vi "Facade.vi"(0 "Data In":T8, 2 "Display State In":T2, 3 "Container State":T7) -> (6 "Data Out":T8, 7 "Display State Out":T2, 8 "Action":T1)   [LabVIEW 2020, in "Interactive Graph.xctl"]
uses:
  Interactive Graph.xctl
  Data.vi
  EPhys/LV Source/Work Panel VIs/Typedefs/EPhysWork-Label Position.ctl
  <vilib>/_xctls/Container State.ctl
  State.vi
  Persistent.ctl
  Plot.ctl
  Events.ctl
  Selection.ctl
  XRange.ctl
  YScale.ctl
  Cursor.ctl
  <vilib>/_xctls/Action.ctl
  Scale Selector/Scale Selector.xctl
  <vilib>/Utility/miscctls.llb/LVAnnotationListTypeDef.ctl
  <vilib>/_xctls/XControlSupport.lvlib
panel:
  in  "Scale":dbl(xcontrol)
  out "Graph":cluster{dbl[], dbl[]}[](graph)
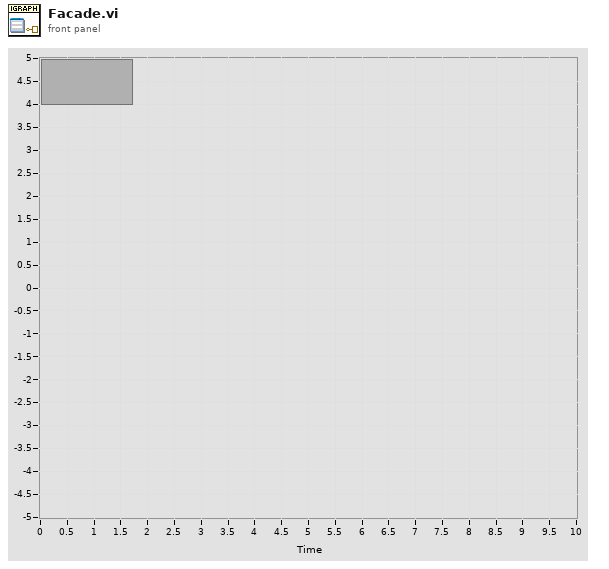
[diagram p1: front panel]
types:
  T1 = typedef "XControlSupport.lvlib/Action.ctl" = cluster{"Data Changed?":bool, "State Changed?":bool, "Action Name":string}
  T2 = typedef "Interactive Graph.xctl/State.vi" = cluster{"ref":refnum<vi>, "actions":string[], "Persist":T3, "cursor":bool, "prescale":dbl, "palette":u32[], "colIndex":i32, "to add":T4, "Events":T6, "selected":i32, "to show":cluster{"Visible":bool, "Start":i32, "Length":i32}, "maxplot":i32, "Y0":dbl[], "plotnum":i32, "length":i32}
  T3 = typedef "Interactive Graph.xctl/Persistent.ctl" = cluster{"Scale":dbl, "Xrange":cluster{"min":dbl, "max":dbl}}
  T4 = typedef "Interactive Graph.xctl/Plot.ctl" = cluster{"plot":cluster{"X":dbl[], "Y":dbl[]}, "name":string, "Y0":dbl, "color":u32, "Style":enum16{"Normal", "Highlight", "Shadow"}, "labpos":T5, "visible":bool, "cursor":bool}
  T5 = typedef "EPhysWork-Label Position.ctl" = cluster{"Index":i32, "Xoff":dbl, "Yoff":dbl}
  T6 = typedef "Interactive Graph.xctl/Events.ctl" = cluster{"Selection":refnum<user-event>, "XRange":refnum<user-event>, "YScale":refnum<user-event>, "CursorPos":refnum<user-event>}
  T7 = typedef "XControlSupport.lvlib/Container State.ctl" = cluster{"Indicator?":bool, "Run Mode?":bool, " Refnum":refnum<vi>}
  T8 = typedef "Interactive Graph.xctl/Data.vi" = cluster{"plot":cluster{"X":dbl[], "Y":dbl[]}, "name":string, "Y0":dbl, "color":u32, "Style":enum16{"Normal", "Highlight", "Shadow"}, "labpos":T5, "visible":bool, "cursor":bool}[]
  T9 = typedef "LVAnnotationListTypeDef.ctl" = cluster{"Name":string, "Color":u32, "Style":u8, "Point Style":u8, "Name Visible":bool, "Allow Drag":bool, "Annotation Mode":u32, "Plot":i32, "Index":i32, "Position":cluster{"X":dbl, "Y":dbl}, "X Scale":u32, "Y Scale":u32, "Show Arrow":bool, "Lock Name":bool, "Plot Area":i32, "Label Offset":cluster{"X":dbl, "Y":dbl}}[]
  T10 = typedef "LVRectTypeDef.ctl" = cluster{"Left":i16, "Top":i16, "Right":i16, "Bottom":i16}
  T11 = typedef "LVPoint32TypeDef.ctl" = cluster{"Horizontal":i32, "Vertical":i32}
  T12 = typedef "PlotDrag-State.ctl" = cluster{"PlotNum":i32, "Y0":dbl, "Plot":cluster{dbl[], dbl[]}, "Drag":bool, "Moved":bool, "dY":dbl, "keyIndex":i32}
  T13 = cluster{"plot":cluster{"X":dbl[], "Y":dbl[]}, "name":string, "Y0":dbl, "color":u32, "Style":enum16{"Normal", "Highlight", "Shadow"}, "labpos":T5, "visible":bool, "cursor":bool}[]
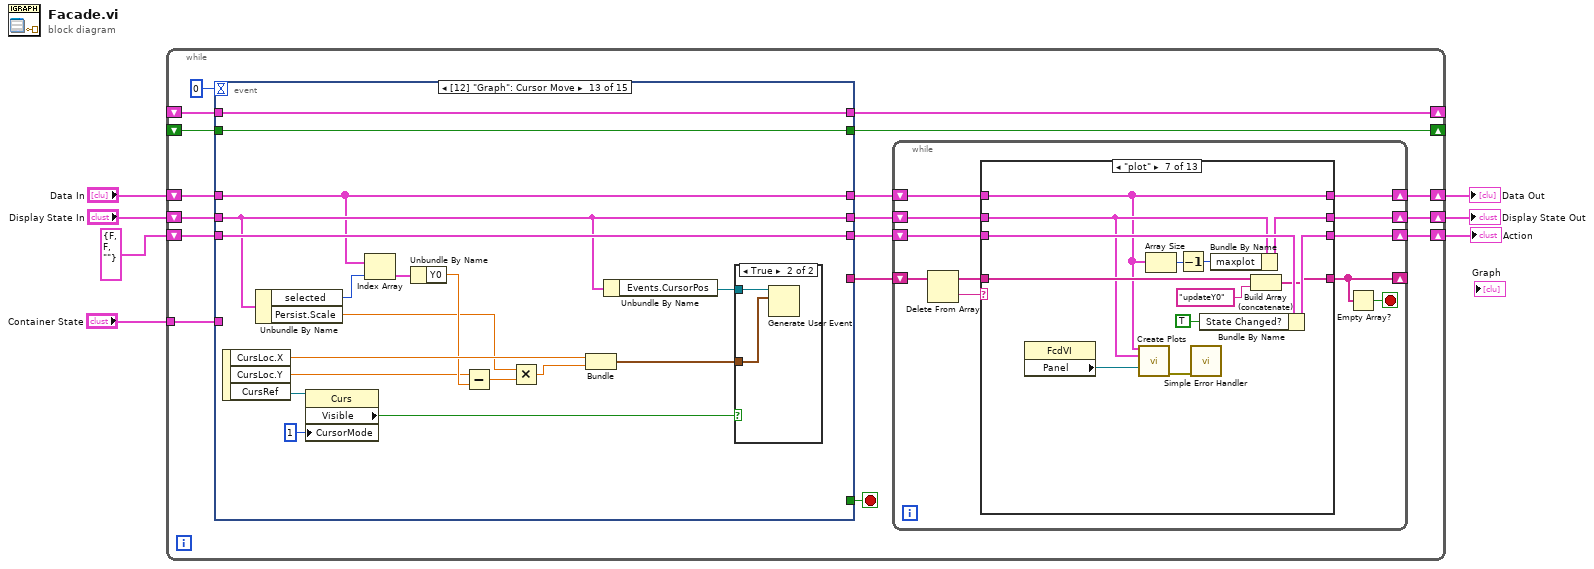
[diagram p0: block diagram]
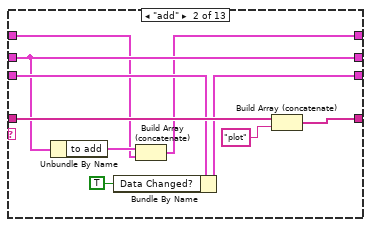
[diagram p3: hidden frame]
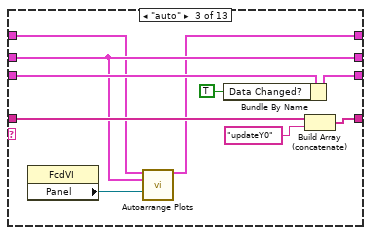
[diagram p4: hidden frame]
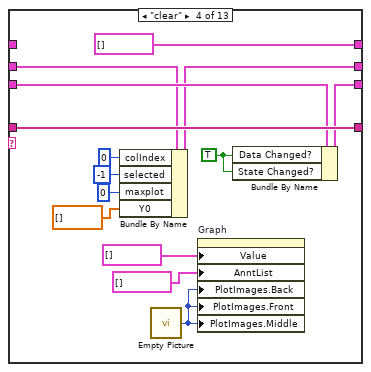
[diagram p5: hidden frame]
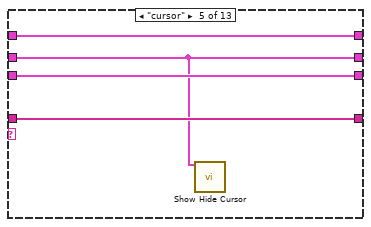
[diagram p6: hidden frame]
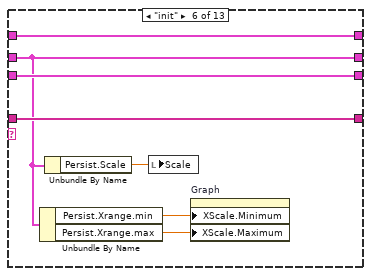
[diagram p7: hidden frame]
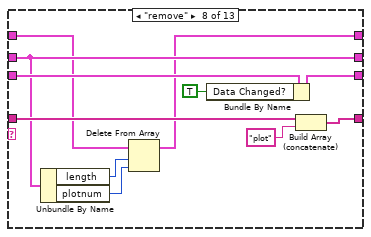
[diagram p8: hidden frame]
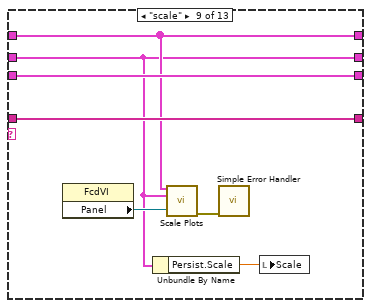
[diagram p9: hidden frame]
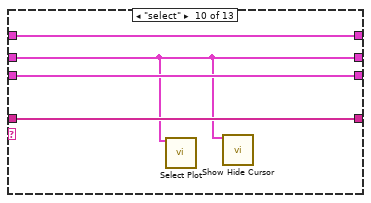
[diagram p10: hidden frame]
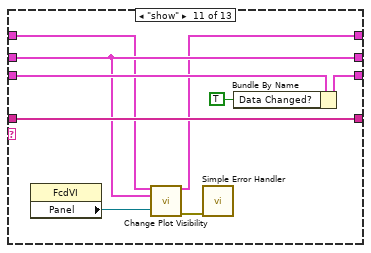
[diagram p11: hidden frame]
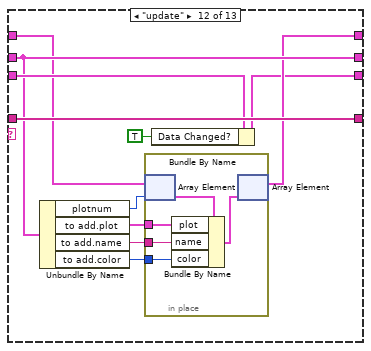
[diagram p12: hidden frame]
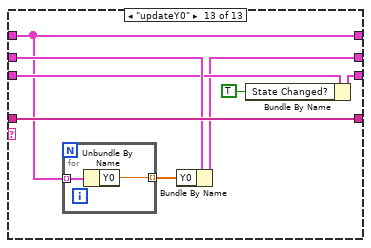
[diagram p13: hidden frame]
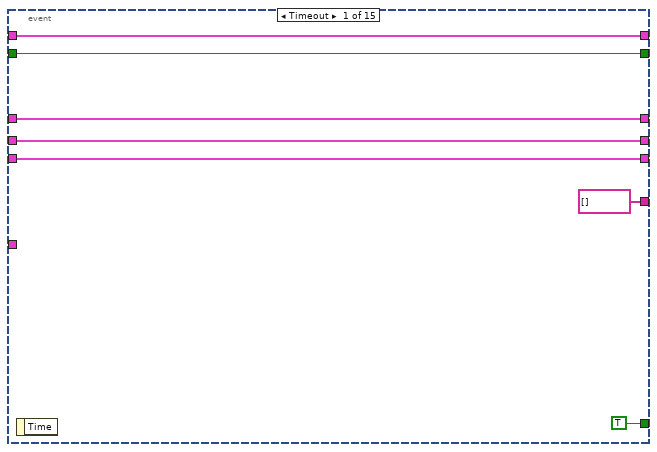
[diagram p14: hidden frame]
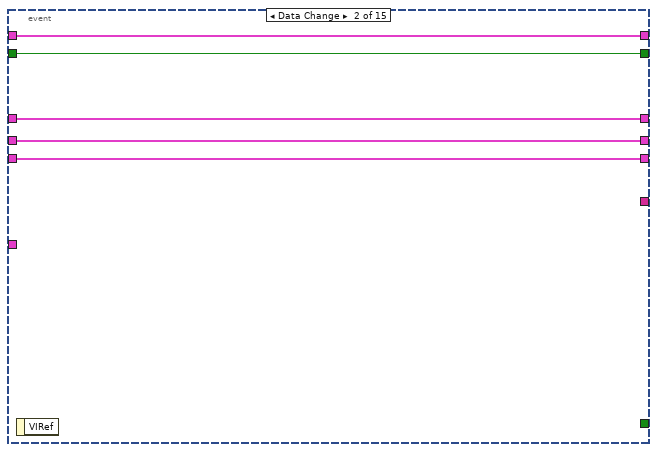
[diagram p15: hidden frame]
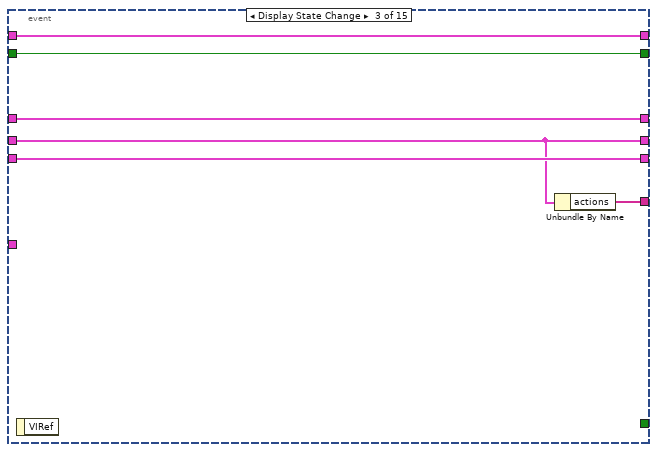
[diagram p16: hidden frame]
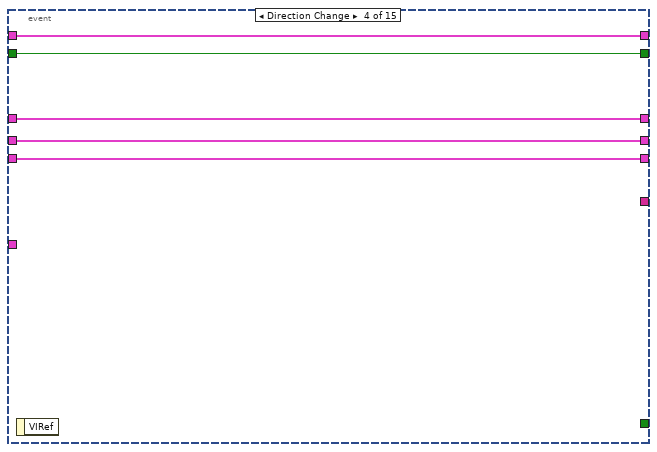
[diagram p17: hidden frame]
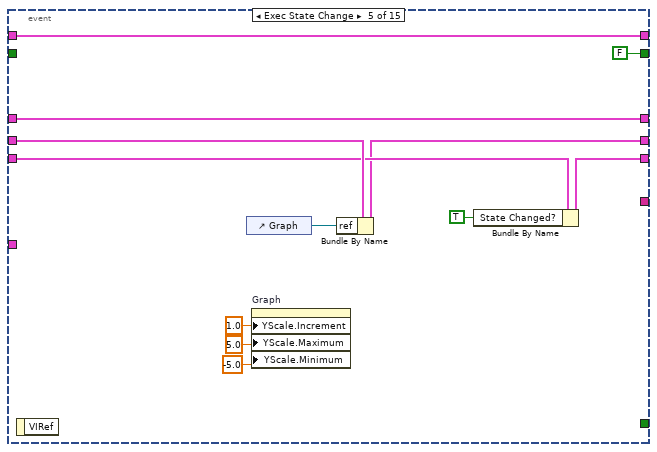
[diagram p18: hidden frame]
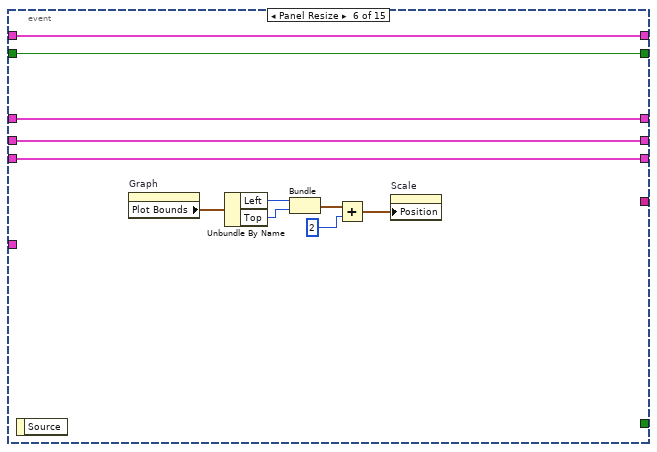
[diagram p19: hidden frame]
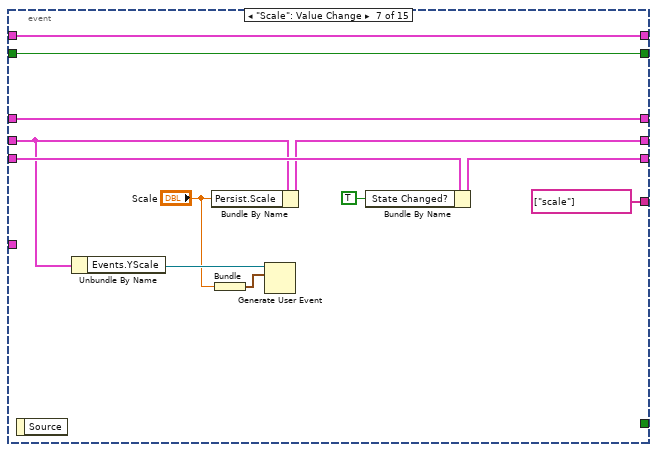
[diagram p20: hidden frame]
diagram:
  n1 = while {
    shift-right: [w14] -> w4
    shift-left: "Display State In" -> [w24]
    tunnel: "Container State" -> [w21]
    shift-right: [w15] -> w7
    shift-left: "Data In" -> [w20]
    shift-right: [w13] -> w2
    shift-left: T1 {"Data Changed?"=FALSE, "State Changed?"=FALSE, "Action Name"=""} ("Action") -> [w19]
    shift-right: [w10] -> _
    shift-left: _ -> [w11]
    shift-right: [w9] -> _
    shift-left: _ -> [w8]
    stop <- w23 stop-if-true
    n2 = event shown="[12] \"Graph\": Cursor Move" {
      selector: _ -> [_ _ _ _ _ _ _ _ _ _ _ _ _ _ _]
      dyn-events: _ -> [_ _ _ _ _ _ _ _ _ _ _ _ _ _ _]
      timeout: 0 -> [_ _ _ _ _ _ _ _ _ _ _ _ _ _ _]
      tunnel: w24 -> [w159 w165 w170 w177 w189 w200 w206 w218 w226 w255 w277 w316 w330 w349 w369]
      tunnel: [w159 w165 w170 w177 w185 w200 w210 w221 w226 w255 w276 w312 w330 w349 w369] -> w17
      tunnel: [TRUE _ _ _ _ _ _ _ _ _ _ _ _ _ _] -> w23
      tunnel: w21 -> [_ _ _ _ _ _ _ _ _ _ w266 _ _ _ w364]
      tunnel: w20 -> [w158 w166 w172 w176 w188 w199 w212 w224 w234 w257 w270 w315 w327 w356 w368]
      tunnel: [w158 w166 w172 w176 w188 w199 w212 w224 w234 w257 w269 w315 w327 w356 w368] -> w18
      tunnel: [w160 w164 w171 w175 w183 w198 w209 w220 w233 w256 w267 w310 w334 w359 w367] -> w16
      tunnel: w19 -> [w160 w164 w171 w175 w187 w198 w211 w223 w233 w256 w268 w314 w334 w359 w367]
      tunnel: [string[] [] _ w169 _ _ _ string[] ["scale"] ("actions") _ _ _ w275 string[] ["select"] ("actions") _ _ _] -> w12
      tunnel: [w156 w163 w168 w174 w181 w191 w207 w222 w230 w252 w280 w313 w333 w344 w366] -> w10
      tunnel: w11 -> [w156 w163 w168 w174 w181 w191 w207 w222 w229 w253 w278 w313 w333 w346 w366]
      tunnel: [w155 w162 w167 w173 FALSE w190 w202 w213 w225 w250 w271 TRUE w331 w358 FALSE] -> w9
      tunnel: w8 -> [w155 w162 w167 w173 _ w190 w202 w213 w225 w250 w271 _ w331 w358 _]
      event Timeout {
        n3 = event-data() -> ()  [unwired: 1 in, 1 out]
      }
      event Data Change {
        n4 = event-data() -> ()  [unwired: 1 in, 1 out]
      }
      event Display State Change {
        n5 = event-data() -> ()  [unwired: 1 in, 1 out]
        n6 = Unbundle By Name(w170) -> ("actions"=w169:string[])
      }
      event Direction Change {
        n7 = event-data() -> ()  [unwired: 1 in, 1 out]
      }
      event Exec State Change {
        n8 = event-data() -> ()  [unwired: 1 in, 1 out]
        n9 = control-ref of="Graph"() -> (w184:refnum<vi>)
        n10 = property on="Graph" class="XYGraph (strict)"("YScale.Increment"=1.0 ("Y Scale.Range:Increment"), "YScale.Maximum"=5.0 ("Y Scale.Range:Maximum"), "YScale.Minimum"=-5.0 ("Y Scale.Range:Minimum")) -> ()  [unwired: 2 in, 2 out]
        n11 = Bundle By Name(cluster=w189, "ref"=w184) -> (w185:T2)
        n12 = Bundle By Name(cluster=w187, "State Changed?"=TRUE) -> (w183:T1)
      }
      event Panel Resize {
        n13 = event-data() -> ()  [unwired: 1 in, 1 out]
        n14 = property on="Graph" class="XYGraph (strict)"() -> ("Plot Bounds"=w197:T10)  [unwired: 2 in, 2 out]
        n15 = Unbundle By Name(w197) -> ("Left"=w196:i16, "Top"=w195:i16)
        n16 = Bundle("Left"=w196, "Top"=w195) -> (w194:cluster{"Left":i16, "Top":i16})  [unwired: 1 in]
        n17 = Add(x=w194, y=2) -> (x+y=w192:cluster{"Left":i32, "Top":i32})
        n18 = property on="Scale" class="Scale Selector (strict)"("Position"=w192) -> ()  [unwired: 2 in, 2 out]
      }
      event "Scale": Value Change {
        n19 = event-data() -> ()  [unwired: 1 in, 1 out]
        n20 = Unbundle By Name(w206) -> ("Events.YScale"=w205:refnum<user-event>)
        n21 = Bundle By Name(cluster=w206, "Persist.Scale"="Scale") -> (w210:T2)
        n22 = Bundle("Scale"="Scale") -> (w203:cluster{"Scale":dbl})  [unwired: 1 in]
        n23 = Generate User Event(user event=w205, event data cluster=w203) -> ()  [unwired: 2 in, 2 out]
        n24 = Bundle By Name(cluster=w211, "State Changed?"=TRUE) -> (w209:T1)
      }
      event "Graph": Scale Range Change {
        n25 = event-data() -> ("NewRange.Minimum"=w215:dbl, "NewRange.Maximum"=w216:dbl)  [unwired: 1 in]
        n26 = Unbundle By Name(w218) -> ("Events.XRange"=w217:refnum<user-event>)
        n27 = Bundle By Name(cluster=w218, "Persist.Xrange.min"=w215, "Persist.Xrange.max"=w216) -> (w221:T2)
        n28 = Bundle("Minimum"=w215, "Maximum"=w216) -> (w214:cluster{"Minimum":dbl, "Maximum":dbl})  [unwired: 1 in]
        n29 = Generate User Event(user event=w217, event data cluster=w214) -> ()  [unwired: 2 in, 2 out]
        n30 = Bundle By Name(cluster=w223, "State Changed?"=TRUE) -> (w220:T1)
      }
      event "Graph": Mouse Down {
        n31 = event-data() -> ("Coords"=w231:T11, "Button"=w227:u16, "PlatMods.Ctrl"=w228:bool)  [unwired: 1 in]
        n32 = Unbundle By Name(w226) -> ("ref"=w232:refnum<vi>)
        n33 = case shown="1" w227 {
          tunnel: w232 -> [_ w241]
          tunnel: w231 -> [_ w240]
          tunnel: [w235 w239] -> w230
          tunnel: w229 -> [w235 w238]
          tunnel: w228 -> [_ w237]
          tunnel: w226 -> [_ w236]
          frame 0, Default {
          }
          frame 1 {
            n34 = case shown="False" w237 {
              tunnel: w241 -> [w242 _]
              tunnel: w240 -> [w245 _]
              tunnel: [w244 w246] -> w239
              tunnel: w238 -> [_ w246]
              tunnel: w236 -> [w243 _]
              frame False {
                n35 = call "Show Hide Cursor.vi"("State"=w243) -> ()  [unwired: 15 in]
                n36 = call "PlotDrag-Mouse Down.vi"("XYGraph ref"=w242, "Coords"=w245) -> ("Drag State"=w244:T12)  [unwired: 11 in, 2 out]
              }
              frame True {
              }
            }
          }
        }
      }
      event "Graph": Mouse Move {
        n37 = event-data() -> ("Coords"=w251:T11)  [unwired: 1 in]
        n38 = Unbundle By Name(w255) -> ("ref"=w254:refnum<vi>)
        n39 = Unbundle By Name(w253) -> ("Drag"=w248:bool)
        n40 = Not(x=w250) -> (.not. x?=w249:bool)
        n41 = And(x=w249, y=w248) -> (x .and. y?=w247:bool)
        n42 = case shown="True" w247 {
          tunnel: w254 -> [_ w263]
          tunnel: w253 -> [w258 w260]
          tunnel: [w258 w262] -> w252
          tunnel: w251 -> [_ w261]
          frame False {
          }
          frame True {
            n43 = Unbundle By Name(w260) -> ("Moved"=w259:bool)
            n44 = call "PlotDrag-Mouse Move.vi"("Drag State In"=w260, "XYGraph in"=w263, "Coords"=w261) -> ("Drag State Out"=w262:T12)  [unwired: 11 in, 1 out]
            n45 = case shown="False" w259 {
              frame False {
                n46 = call "Empty Picture"() -> ("empty picture"=w264:picture)
                n47 = property on="Graph" class="XYGraph (strict)"("PlotImages.Middle"=w264, "PlotImages.Back"=w264, "PlotImages.Front"=w264) -> ()  [unwired: 2 in, 2 out]
              }
              frame True {
              }
            }
          }
        }
      }
      event "Graph": Mouse Up {
        n48 = event-data() -> ()  [unwired: 1 in, 1 out]
        n49 = Unbundle By Name(w266) -> ("Refnum"=w265:refnum<vi>)
        n50 = Unbundle By Name(w278) -> ("Drag"=w273:bool)
        n51 = Not(x=w271) -> (.not. x?=w272:bool)
        n52 = And(x=w272, y=w273) -> (x .and. y?=w274:bool)
        n53 = case shown="True" w274 {
          tunnel: w277 -> [w283 w296]
          tunnel: w278 -> [_ w304]
          tunnel: [w283 w303] -> w276
          tunnel: [_ string[] ["cursor", "updateY0"]] -> w275
          tunnel: w270 -> [w282 w299]
          tunnel: [w282 w298] -> w269
          tunnel: w268 -> [w281 w292]
          tunnel: [w281 w293] -> w267
          tunnel: w265 -> [_ w284]
          frame False {
          }
          frame True {
            w294 = TRUE
            n54 = Unbundle By Name(w304) -> ("dY"=w301:dbl, "PlotNum"=w287:i32)
            n55 = Unbundle By Name(w296) -> ("maxplot"=w295:i32)
            n56 = property class="Ctl"(reference=w284, "Key Focus"=TRUE) -> ()  [unwired: 1 in, 2 out]
            n57 = Unbundle By Name(w296) -> ("Events.Selection"=w306:refnum<user-event>)
            n58 = Index Array(array=w299, index=w287) -> (element=w291:T4)
            n59 = Subtract(x=w295, y=w287) -> (x-y=w288:i32)
            n60 = Greater Or Equal To 0?(x=w287) -> (x >= 0?=w289:bool)
            n61 = Unbundle By Name(w291) -> ("Y0"=w290:dbl)
            n62 = Bundle By Name(cluster=w296, "selected"=w287) -> (w303:T2)
            n63 = Select(t=w288, s=w289, f=w287) -> (s? t:f=w286:i32)
            n64 = Add(x=w290, y=w301) -> (x+y=w300:dbl)
            n65 = Bundle("PlotNum"=w286) -> (w305:cluster{"PlotNum":i32})  [unwired: 1 in]
            n66 = Bundle By Name(cluster=w292, "Data Changed?"=w294, "State Changed?"=w294) -> (w293:T1)
            n67 = Bundle By Name(cluster=w291, "Y0"=w300) -> (w297:T4)
            n68 = Generate User Event(user event=w306, event data cluster=w305) -> ()  [unwired: 2 in, 2 out]
            n69 = Replace Array Subset(array=w299, new element=w297, index=w287) -> (w298:T4[])
          }
        }
        n70 = Bundle By Name(cluster=w278, "Drag"=FALSE) -> (w280:T12)
      }
      event "Graph": Cursor Grab {
        n71 = event-data() -> ("PlotIdx"=w311:i32)  [unwired: 1 in]
        n72 = Bundle By Name(cluster=w316, "selected"=w311) -> (w312:T2)
        n73 = Bundle By Name(cluster=w314, "State Changed?"=TRUE) -> (w310:T1)
      }
      event "Graph": Cursor Move {
        n74 = event-data() -> ("CursLoc.X"=w329:dbl, "CursLoc.Y"=w323:dbl, "CursRef"=w319:refnum<vi>)  [unwired: 1 in]
        n75 = Unbundle By Name(w330) -> ("selected"=w326:i32, "Persist.Scale"=w321:dbl)
        n76 = property class="Curs"(reference=w319, "CursorMode"=u32 1 ("Cursor Mode")) -> ("Visible"=w318:bool)  [unwired: 1 in, 2 out]
        n77 = Index Array(array=w327, index=w326) -> (element=w325:T4)
        n78 = Unbundle By Name(w325) -> ("Y0"=w324:dbl)
        n79 = Subtract(x=w323, y=w324) -> (x-y=w322:dbl)
        n80 = Multiply(x=w321, y=w322) -> (x*y=w320:dbl)
        n81 = Bundle("X"=w329, w320) -> (w328:cluster{"X":dbl, dbl})  [unwired: 1 in]
        n82 = Unbundle By Name(w330) -> ("Events.CursorPos"=w332:refnum<user-event>)
        n83 = case shown="True" w318 {
          tunnel: w332 -> [_ w336]
          tunnel: w328 -> [_ w335]
          frame False {
          }
          frame True {
            n84 = Generate User Event(user event=w336, event data cluster=w335) -> ()  [unwired: 2 in, 2 out]
          }
        }
      }
      event Key Up {
        n85 = event-data() -> ("ScanCode"=w342:i16, "PlatMods.Ctrl"=w341:bool)  [unwired: 1 in]
        n86 = Unbundle By Name(w349) -> ("selected"=w337:i32)
        n87 = Index Array(array=w356, index=w337) -> (element=w357:T4)
        n88 = Unbundle By Name(w346) -> ("keyIndex"=w345:i32)
        n89 = Unbundle By Name(w349) -> ("Persist.Scale"=w340:dbl)
        n90 = control-ref of="Graph"() -> (w355:refnum<vi>)
        n91 = Unbundle By Name(w357) -> ("Y0"=w339:dbl, "plot.X"=w338:dbl[])
        n92 = call "Move Cursor With Keys.vi"("XYGraph in"=w355, "index in"=w345, "X"=w338, "plotIndex"=w337, "ScanCode"=w342, "Control?"=w341) -> ("index out"=w343:i32, "X"=w351:dbl, "Y"=w352:dbl, "moved"=w347:bool)  [unwired: 6 in]
        n93 = Subtract(x=w352, y=w339) -> (x-y=w354:dbl)
        n94 = Bundle By Name(cluster=w346, "keyIndex"=w343) -> (w344:T12)
        n95 = Multiply(x=w340, y=w354) -> (x*y=w353:dbl)
        n96 = Unbundle By Name(w349) -> ("Events.CursorPos"=w350:refnum<user-event>)
        n97 = Bundle("X"=w351, w353) -> (w348:cluster{"X":dbl, dbl})  [unwired: 1 in]
        n98 = case shown="True" w347 {
          tunnel: w350 -> [_ w361]
          tunnel: w348 -> [_ w360]
          frame False {
          }
          frame True {
            n99 = Generate User Event(user event=w361, event data cluster=w360) -> ()  [unwired: 2 in, 2 out]
          }
        }
      }
      event "Graph": Cursor Release {
        n100 = event-data() -> ()  [unwired: 1 in, 1 out]
        n101 = Unbundle By Name(w364) -> ("Refnum"=w363:refnum<vi>)
        n102 = property class="Ctl"(reference=w363, "Key Focus"=TRUE) -> ()  [unwired: 1 in, 2 out]
      }
    }
    n103 = while {
      shift-right: [w32] -> _
      shift-left: w12 -> [w35]
      shift-right: [w25] -> w13
      shift-left: w16 -> [w28]
      shift-right: [w26] -> w14
      shift-left: w17 -> [w29]
      shift-right: [w27] -> w15
      shift-left: w18 -> [w30]
      stop <- w31 stop-if-true
      n104 = Delete From Array(array=w35) -> (deleted portion=w33:string, array with subset deleted=w34:string[])  [unwired: 2 in]
      n105 = case shown="\"plot\"" w33 {
        tunnel: w34 -> [w39 w49 w59 w73 w77 w84 w97 w108 w115 w119 w128 w139 w152]
        tunnel: [w39 w43 w55 w73 w77 w84 w86 w99 w115 w119 w128 w139 w152] -> w32
        tunnel: w30 -> [w38 w40 w53 _ w76 w83 w92 w103 w112 w118 w123 w132 w149]
        tunnel: w29 -> [w37 w47 w56 w70 w74 w80 w95 w106 w110 w116 w126 w137 w151]
        tunnel: w28 -> [w36 w48 w58 w72 w75 w82 w96 w107 w114 w117 w127 w138 w150]
        tunnel: [w38 w46 w52 T8 [] ("Data out") w76 w83 w92 w102 w112 w118 w122 w131 w149] -> w27
        tunnel: [w37 w47 w56 w67 w74 w80 w91 w106 w110 w116 w126 w137 w148] -> w26
        tunnel: [w36 w45 w51 w71 w75 w82 w89 w101 w114 w117 w121 w130 w146] -> w25
        frame "", Default {
        }
        frame "add" {
          n106 = Unbundle By Name(w47) -> ("to add"=w41:T4)
          n107 = Bundle By Name(cluster=w48, "Data Changed?"=TRUE) -> (w45:T1)
          n108 = Build Array (concatenate)(w41, w40) -> (w46:T4[])
          n109 = Build Array (concatenate)(w49, "plot") -> (w43:string[])
        }
        frame "auto" {
          n110 = property class="FcdVI"() -> ("Panel"=w57:refnum<vi>)  [unwired: 2 in, 2 out]
          n111 = call "Autoarrange Plots.vi"("Data in"=w53, "Display State"=w56, "panel"=w57) -> ("Data out"=w52:T13)  [unwired: 11 in, 1 out]
          n112 = Bundle By Name(cluster=w58, "Data Changed?"=TRUE) -> (w51:T1)
          n113 = Build Array (concatenate)(w59, "updateY0") -> (w55:string[])
        }
        frame "clear" {
          w68 = TRUE ("Data Changed?")
          n114 = Bundle By Name(cluster=w70, "colIndex"=0, "selected"=-1, "maxplot"=0 ("Nplot"), "Y0"=dbl[] []) -> (w67:T2)
          n115 = call "Empty Picture"() -> ("empty picture"=w60:picture)
          n116 = property on="Graph" class="XYGraph (strict)"("Value"=cluster{dbl[], dbl[]}[] [] ("Graph"), "AnntList"=T9 [] ("Annotation List"), "PlotImages.Back"=w60, "PlotImages.Front"=w60, "PlotImages.Middle"=w60) -> ()  [unwired: 2 in, 2 out]
          n117 = Bundle By Name(cluster=w72, "Data Changed?"=w68, "State Changed?"=w68) -> (w71:T1)
        }
        frame "cursor" {
          n118 = call "Show Hide Cursor.vi"("State"=w74) -> ()  [unwired: 15 in]
        }
        frame "init" {
          n119 = Unbundle By Name(w80) -> ("Persist.Xrange.min"=w79:dbl, "Persist.Xrange.max"=w78:dbl)
          n120 = Unbundle By Name(w80) -> ("Persist.Scale"=w81:dbl)
          n121 = local write "Scale"(w81) -> ()
          n122 = property on="Graph" class="XYGraph (strict)"("XScale.Minimum"=w79, "XScale.Maximum"=w78) -> ()  [unwired: 2 in, 2 out]
        }
        frame "plot" {
          n123 = property class="FcdVI"() -> ("Panel"=w93:refnum<vi>)  [unwired: 2 in, 2 out]
          n124 = call "Create Plots.vi"("Data in"=w92, "Display State"=w95, "panel"=w93) -> ("error out"=w94:errorcluster)  [unwired: 12 in]
          n125 = Array Size(array=w92) -> (size(s)=w90:i32)
          n126 = Decrement(x=w90) -> (x-1=w87:i32)
          n127 = call <vilib>:"Simple Error Handler.vi"("error in (no error)"=w94) -> ()  [unwired: 4 in, 5 out]
          n128 = Bundle By Name(cluster=w96, "State Changed?"=TRUE) -> (w89:T1)
          n129 = Bundle By Name(cluster=w95, "maxplot"=w87) -> (w91:T2)
          n130 = Build Array (concatenate)(w97, "updateY0") -> (w86:string[])
        }
        frame "remove" {
          n131 = Unbundle By Name(w106) -> ("length"=w105:i32, "plotnum"=w104:i32)
          n132 = Delete From Array(array=w103, length=w105, index=w104) -> (array with subset deleted=w102:T4[])  [unwired: 1 out]
          n133 = Bundle By Name(cluster=w107, "Data Changed?"=TRUE) -> (w101:T1)
          n134 = Build Array (concatenate)(w108, "plot") -> (w99:string[])
        }
        frame "scale" {
          n135 = property class="FcdVI"() -> ("Panel"=w111:refnum<vi>)  [unwired: 2 in, 2 out]
          n136 = Unbundle By Name(w110) -> ("Persist.Scale"=w109:dbl)
          n137 = call "Scale Plots.vi"("Data in"=w112, "Display State"=w110, "panel"=w111) -> ("error out"=w113:errorcluster)  [unwired: 12 in]
          n138 = call <vilib>:"Simple Error Handler.vi"("error in (no error)"=w113) -> ()  [unwired: 4 in, 5 out]
          n139 = local write "Scale"(w109) -> ()
        }
        frame "select" {
          n140 = call "Select Plot.vi"("State"=w116) -> ()  [unwired: 15 in]
          n141 = call "Show Hide Cursor.vi"("State"=w116) -> ()  [unwired: 15 in]
        }
        frame "show" {
          n142 = property class="FcdVI"() -> ("Panel"=w124:refnum<vi>)  [unwired: 2 in, 2 out]
          n143 = call "Change Plot Visibility.vi"("Data in"=w123, "Display State"=w126, "panel"=w124) -> ("Data out"=w122:T8, "error out"=w125:errorcluster)  [unwired: 11 in]
          n144 = call <vilib>:"Simple Error Handler.vi"("error in (no error)"=w125) -> ()  [unwired: 4 in, 5 out]
          n145 = Bundle By Name(cluster=w127, "Data Changed?"=TRUE) -> (w121:T1)
        }
        frame "update" {
          n146 = Unbundle By Name(w137) -> ("plotnum"=w136:i32, "to add.plot"=w135:cluster{"X":dbl[], "Y":dbl[]}, "to add.name"=w134:string, "to add.color"=w133:u32)
          n147 = in-place {
            in-place-border: w135 -> [w142]
            in-place-border: w134 -> [w141]
            in-place-border: w133 -> [w140]
            n148 = in-place-array #1(w132, w136) -> (w144:T4)
            n149 = Bundle By Name(cluster=w144, "plot"=w142, "name"=w141, "color"=w140) -> (w143:T4)
            n150 = in-place-array #1(w143) -> (w131:T4[])  [unwired: 1 out]
          }
          n151 = Bundle By Name(cluster=w138, "Data Changed?"=TRUE) -> (w130:T1)
        }
        frame "updateY0" {
          n152 = for {
            tunnel: w149 -> [w154] mode=indexing
            tunnel: [w153] -> w147 mode=indexing
            n153 = Unbundle By Name(w154) -> ("Y0"=w153:dbl)
          }
          n154 = Bundle By Name(cluster=w151, "Y0"=w147) -> (w148:T2)
          n155 = Bundle By Name(cluster=w150, "State Changed?"=TRUE) -> (w146:T1)
        }
      }
      n156 = Empty Array?(array=w32) -> (empty?=w31:bool)
    }
  }
  "Display State Out" <- w4
  "Data Out" <- w7
  "Action" <- w2
